vi "disc.vi"(1 "c":dbl, 2 "b":dbl, 3 "a":dbl) -> (0 "discOut":dbl)   [LabVIEW 2019]
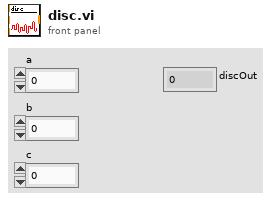
[diagram p1: front panel]
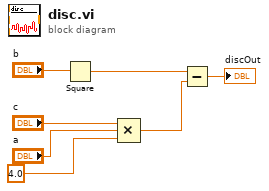
[diagram p0: block diagram]
diagram:
  n1 = Square(x="b") -> (x^2=w6:dbl)
  n2 = Compound Arithmetic op=MULTIPLY("c", "a", 4.0) -> (w2:dbl)
  n3 = Subtract(x=w6, y=w2) -> (x-y=→"discOut":dbl)
